vi "Write Log Session.vi"(8 "error in":errorcluster, 10 "Session Handle":T1, 11 "Ex Nested in":refnum<class "SuperActor.lvclass">) -> (0 "error out":errorcluster, 3 "Ex Nested out":refnum<class "SuperActor.lvclass">)   [LabVIEW 2015, in "SuperActor.lvclass"]
uses:
  SuperActor.lvclass
  <vilib>/MSR Consulting, LLC/General Reuse/Session APIs/_Session Fwk/Typedefs/Session Handle.ctl
  <vilib>/MSR Consulting, LLC/General Reuse/Session APIs/_Session Fwk/Session - Root.lvclass
  SuperActor.lvclass/SuperActor.ctl
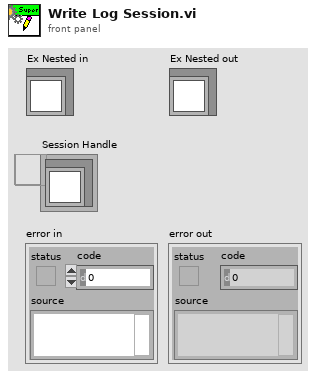
[diagram p1: front panel]
types:
  T1 = typedef "Session - Root.lvclass/Session Handle.ctl" = refnum<data-value>
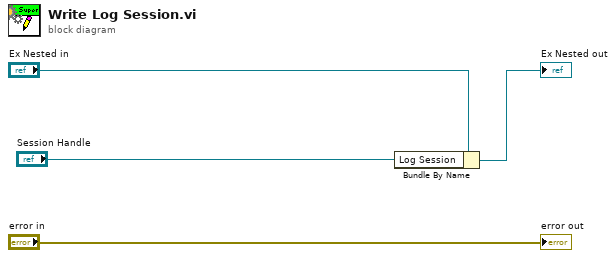
[diagram p0: block diagram]
diagram:
  n1 = Bundle By Name(cluster="Ex Nested in", "Log Session"="Session Handle") -> (→"Ex Nested out":refnum<class "SuperActor.lvclass">)
  "error out" <- "error in"
